vi "SPAN LIN speichern Parameter bestimmern.vi"(11 "SpanInletClusterArray out (Eingang)":T1[](array[typedef]) {"zusätzliche Zeitdauer Erster Punkt" min=30 step=1 format="%#_5g"; "Zeitdauer Stufen" format="%#_5g"; "Max Fehler" format="%#_5g"; "Anzahl Stufen" format="%#_5g"; "Komponenten"."Komponente 5"."Komponente:" items=["NO (350,3000) LP 191C", "NO2 (150) LP 191C (1of2)", "NO2 (2000) LP 191C (2of2)", "N2O (300) LP 191C (1of2)", "NH3 (300) LP 191C (1of2)", "NH3 (900,3000) LP 191C (2of2)", "HNCO (400) 191C", "H2O% (30) LP 191C", "Formaldehyde (70,500) LP 191C", "CO2 low% (4) LP 191C (2of2)", "CO2% (20) LP 191C (1of2)", "CO (700) LP 191C (1of3)", "CO% (1) LP 191C (2of3)", "Propylene (1000) LP 191C", "Aromatic HC C7 (500) LP 191C", "Ethylene (1000) LP 191C", "CH4 (250) LP 191C (1of2)", "CH4 (5000) LP 191C (2of2)", "Ethane (1000) LP 191C", "Acetylene (1000) LP 191C", "HNO2 (20) 191C", "MeOH (1000) 191C", "CO% (10) LP 191C (3of3)", "Formic Acid (100) 191C", "SO2 (500) LP 191C", "Acetaldehyde (1000) LP 191C", "COS (100) LP 191C", "1,3 butadiene (100) LP 191C", "Oil as Octane (200) LP 191C", "N2O (1000) LP 191C (2of2)", "Propane (200) LP 191C", "NO2 autorange (2000)", "CO autorange (100000)", "CH4 autorange (5000)", "NH3 autorange (3000)", "Temp. Gascell", "Pressure Gascell", "sBeam@2500"]; "Komponenten"."Komponente 5"."Konzentration IST" format="%#.4f"; "Komponenten"."Komponente 5"."Genauigkeit" format="%#.1f"; "Komponenten"."Komponente 4"."Komponente:" items=["NO (350,3000) LP 191C", "NO2 (150) LP 191C (1of2)", "NO2 (2000) LP 191C (2of2)", "N2O (300) LP 191C (1of2)", "NH3 (300) LP 191C (1of2)", "NH3 (900,3000) LP 191C (2of2)", "HNCO (400) 191C", "H2O% (30) LP 191C", "Formaldehyde (70,500) LP 191C", "CO2 low% (4) LP 191C (2of2)", "CO2% (20) LP 191C (1of2)", "CO (700) LP 191C (1of3)", "CO% (1) LP 191C (2of3)", "Propylene (1000) LP 191C", "Aromatic HC C7 (500) LP 191C", "Ethylene (1000) LP 191C", "CH4 (250) LP 191C (1of2)", "CH4 (5000) LP 191C (2of2)", "Ethane (1000) LP 191C", "Acetylene (1000) LP 191C", "HNO2 (20) 191C", "MeOH (1000) 191C", "CO% (10) LP 191C (3of3)", "Formic Acid (100) 191C", "SO2 (500) LP 191C", "Acetaldehyde (1000) LP 191C", "COS (100) LP 191C", "1,3 butadiene (100) LP 191C", "Oil as Octane (200) LP 191C", "N2O (1000) LP 191C (2of2)", "Propane (200) LP 191C", "NO2 autorange (2000)", "CO autorange (100000)", "CH4 autorange (5000)", "NH3 autorange (3000)", "Temp. Gascell", "Pressure Gascell", "sBeam@2500"]; "Komponenten"."Komponente 4"."Konzentration IST" format="%#.4f"; "Komponenten"."Komponente 4"."Genauigkeit" format="%#.1f"; "Komponenten"."Komponente 3"."Komponente:" items=["NO (350,3000) LP 191C", "NO2 (150) LP 191C (1of2)", "NO2 (2000) LP 191C (2of2)", "N2O (300) LP 191C (1of2)", "NH3 (300) LP 191C (1of2)", "NH3 (900,3000) LP 191C (2of2)", "HNCO (400) 191C", "H2O% (30) LP 191C", "Formaldehyde (70,500) LP 191C", "CO2 low% (4) LP 191C (2of2)", "CO2% (20) LP 191C (1of2)", "CO (700) LP 191C (1of3)", "CO% (1) LP 191C (2of3)", "Propylene (1000) LP 191C", "Aromatic HC C7 (500) LP 191C", "Ethylene (1000) LP 191C", "CH4 (250) LP 191C (1of2)", "CH4 (5000) LP 191C (2of2)", "Ethane (1000) LP 191C", "Acetylene (1000) LP 191C", "HNO2 (20) 191C", "MeOH (1000) 191C", "CO% (10) LP 191C (3of3)", "Formic Acid (100) 191C", "SO2 (500) LP 191C", "Acetaldehyde (1000) LP 191C", "COS (100) LP 191C", "1,3 butadiene (100) LP 191C", "Oil as Octane (200) LP 191C", "N2O (1000) LP 191C (2of2)", "Propane (200) LP 191C", "NO2 autorange (2000)", "CO autorange (100000)", "CH4 autorange (5000)", "NH3 autorange (3000)", "Temp. Gascell", "Pressure Gascell", "sBeam@2500"]; "Komponenten"."Komponente 3"."Konzentration IST" format="%#.4f"; "Komponenten"."Komponente 3"."Genauigkeit" format="%#.1f"; "Komponenten"."Komponente 2"."Komponente:" items=["NO (350,3000) LP 191C", "NO2 (150) LP 191C (1of2)", "NO2 (2000) LP 191C (2of2)", "N2O (300) LP 191C (1of2)", "NH3 (300) LP 191C (1of2)", "NH3 (900,3000) LP 191C (2of2)", "HNCO (400) 191C", "H2O% (30) LP 191C", "Formaldehyde (70,500) LP 191C", "CO2 low% (4) LP 191C (2of2)", "CO2% (20) LP 191C (1of2)", "CO (700) LP 191C (1of3)", "CO% (1) LP 191C (2of3)", "Propylene (1000) LP 191C", "Aromatic HC C7 (500) LP 191C", "Ethylene (1000) LP 191C", "CH4 (250) LP 191C (1of2)", "CH4 (5000) LP 191C (2of2)", "Ethane (1000) LP 191C", "Acetylene (1000) LP 191C", "HNO2 (20) 191C", "MeOH (1000) 191C", "CO% (10) LP 191C (3of3)", "Formic Acid (100) 191C", "SO2 (500) LP 191C", "Acetaldehyde (1000) LP 191C", "COS (100) LP 191C", "1,3 butadiene (100) LP 191C", "Oil as Octane (200) LP 191C", "N2O (1000) LP 191C (2of2)", "Propane (200) LP 191C", "NO2 autorange (2000)", "CO autorange (100000)", "CH4 autorange (5000)", "NH3 autorange (3000)", "Temp. Gascell", "Pressure Gascell", "sBeam@2500"]; "Komponenten"."Komponente 2"."Konzentration IST" format="%#.4f"; "Komponenten"."Komponente 2"."Genauigkeit" format="%#.1f"; "Komponenten"."Komponente 1"."Komponente:" items=["NO (350,3000) LP 191C", "NO2 (150) LP 191C (1of2)", "NO2 (2000) LP 191C (2of2)", "N2O (300) LP 191C (1of2)", "NH3 (300) LP 191C (1of2)", "NH3 (900,3000) LP 191C (2of2)", "HNCO (400) 191C", "H2O% (30) LP 191C", "Formaldehyde (70,500) LP 191C", "CO2 low% (4) LP 191C (2of2)", "CO2% (20) LP 191C (1of2)", "CO (700) LP 191C (1of3)", "CO% (1) LP 191C (2of3)", "Propylene (1000) LP 191C", "Aromatic HC C7 (500) LP 191C", "Ethylene (1000) LP 191C", "CH4 (250) LP 191C (1of2)", "CH4 (5000) LP 191C (2of2)", "Ethane (1000) LP 191C", "Acetylene (1000) LP 191C", "HNO2 (20) 191C", "MeOH (1000) 191C", "CO% (10) LP 191C (3of3)", "Formic Acid (100) 191C", "SO2 (500) LP 191C", "Acetaldehyde (1000) LP 191C", "COS (100) LP 191C", "1,3 butadiene (100) LP 191C", "Oil as Octane (200) LP 191C", "N2O (1000) LP 191C (2of2)", "Propane (200) LP 191C", "NO2 autorange (2000)", "CO autorange (100000)", "CH4 autorange (5000)", "NH3 autorange (3000)", "Temp. Gascell", "Pressure Gascell", "sBeam@2500"]; "Komponenten"."Komponente 1"."Konzentration IST" format="%#.4f"; "Komponenten"."Komponente 1"."Genauigkeit" format="%#.1f"; "Ablaufdatum" format="%<%d.%m.%Y>T"; "Gasflasche" items=["----"=10000, "IAG NH3 3000"=0, "IAG NH3 200"=1, "IAG NH3 2000"=2, "IAG MG"=3, "IAG O2"=4]}) -> (0 "Anzahl Komponenten OK":bool, 1 "gültige aktiver auto SPAN Index":bool, 2 "Anzahl aktive Komponenten out":i32, 3 "SpanInletClusterArray out (Ausgang)":T1[](array[typedef]) {"zusätzliche Zeitdauer Erster Punkt" min=30 step=1 format="%#_5g"; "Zeitdauer Stufen" format="%#_5g"; "Max Fehler" format="%#_5g"; "Anzahl Stufen" format="%#_5g"; "Komponenten"."Komponente 5"."Komponente:" items=["NO (350,3000) LP 191C", "NO2 (150) LP 191C (1of2)", "NO2 (2000) LP 191C (2of2)", "N2O (300) LP 191C (1of2)", "NH3 (300) LP 191C (1of2)", "NH3 (900,3000) LP 191C (2of2)", "HNCO (400) 191C", "H2O% (30) LP 191C", "Formaldehyde (70,500) LP 191C", "CO2 low% (4) LP 191C (2of2)", "CO2% (20) LP 191C (1of2)", "CO (700) LP 191C (1of3)", "CO% (1) LP 191C (2of3)", "Propylene (1000) LP 191C", "Aromatic HC C7 (500) LP 191C", "Ethylene (1000) LP 191C", "CH4 (250) LP 191C (1of2)", "CH4 (5000) LP 191C (2of2)", "Ethane (1000) LP 191C", "Acetylene (1000) LP 191C", "HNO2 (20) 191C", "MeOH (1000) 191C", "CO% (10) LP 191C (3of3)", "Formic Acid (100) 191C", "SO2 (500) LP 191C", "Acetaldehyde (1000) LP 191C", "COS (100) LP 191C", "1,3 butadiene (100) LP 191C", "Oil as Octane (200) LP 191C", "N2O (1000) LP 191C (2of2)", "Propane (200) LP 191C", "NO2 autorange (2000)", "CO autorange (100000)", "CH4 autorange (5000)", "NH3 autorange (3000)", "Temp. Gascell", "Pressure Gascell", "sBeam@2500"]; "Komponenten"."Komponente 5"."Konzentration IST" format="%#.4f"; "Komponenten"."Komponente 5"."Genauigkeit" format="%#.1f"; "Komponenten"."Komponente 4"."Komponente:" items=["NO (350,3000) LP 191C", "NO2 (150) LP 191C (1of2)", "NO2 (2000) LP 191C (2of2)", "N2O (300) LP 191C (1of2)", "NH3 (300) LP 191C (1of2)", "NH3 (900,3000) LP 191C (2of2)", "HNCO (400) 191C", "H2O% (30) LP 191C", "Formaldehyde (70,500) LP 191C", "CO2 low% (4) LP 191C (2of2)", "CO2% (20) LP 191C (1of2)", "CO (700) LP 191C (1of3)", "CO% (1) LP 191C (2of3)", "Propylene (1000) LP 191C", "Aromatic HC C7 (500) LP 191C", "Ethylene (1000) LP 191C", "CH4 (250) LP 191C (1of2)", "CH4 (5000) LP 191C (2of2)", "Ethane (1000) LP 191C", "Acetylene (1000) LP 191C", "HNO2 (20) 191C", "MeOH (1000) 191C", "CO% (10) LP 191C (3of3)", "Formic Acid (100) 191C", "SO2 (500) LP 191C", "Acetaldehyde (1000) LP 191C", "COS (100) LP 191C", "1,3 butadiene (100) LP 191C", "Oil as Octane (200) LP 191C", "N2O (1000) LP 191C (2of2)", "Propane (200) LP 191C", "NO2 autorange (2000)", "CO autorange (100000)", "CH4 autorange (5000)", "NH3 autorange (3000)", "Temp. Gascell", "Pressure Gascell", "sBeam@2500"]; "Komponenten"."Komponente 4"."Konzentration IST" format="%#.4f"; "Komponenten"."Komponente 4"."Genauigkeit" format="%#.1f"; "Komponenten"."Komponente 3"."Komponente:" items=["NO (350,3000) LP 191C", "NO2 (150) LP 191C (1of2)", "NO2 (2000) LP 191C (2of2)", "N2O (300) LP 191C (1of2)", "NH3 (300) LP 191C (1of2)", "NH3 (900,3000) LP 191C (2of2)", "HNCO (400) 191C", "H2O% (30) LP 191C", "Formaldehyde (70,500) LP 191C", "CO2 low% (4) LP 191C (2of2)", "CO2% (20) LP 191C (1of2)", "CO (700) LP 191C (1of3)", "CO% (1) LP 191C (2of3)", "Propylene (1000) LP 191C", "Aromatic HC C7 (500) LP 191C", "Ethylene (1000) LP 191C", "CH4 (250) LP 191C (1of2)", "CH4 (5000) LP 191C (2of2)", "Ethane (1000) LP 191C", "Acetylene (1000) LP 191C", "HNO2 (20) 191C", "MeOH (1000) 191C", "CO% (10) LP 191C (3of3)", "Formic Acid (100) 191C", "SO2 (500) LP 191C", "Acetaldehyde (1000) LP 191C", "COS (100) LP 191C", "1,3 butadiene (100) LP 191C", "Oil as Octane (200) LP 191C", "N2O (1000) LP 191C (2of2)", "Propane (200) LP 191C", "NO2 autorange (2000)", "CO autorange (100000)", "CH4 autorange (5000)", "NH3 autorange (3000)", "Temp. Gascell", "Pressure Gascell", "sBeam@2500"]; "Komponenten"."Komponente 3"."Konzentration IST" format="%#.4f"; "Komponenten"."Komponente 3"."Genauigkeit" format="%#.1f"; "Komponenten"."Komponente 2"."Komponente:" items=["NO (350,3000) LP 191C", "NO2 (150) LP 191C (1of2)", "NO2 (2000) LP 191C (2of2)", "N2O (300) LP 191C (1of2)", "NH3 (300) LP 191C (1of2)", "NH3 (900,3000) LP 191C (2of2)", "HNCO (400) 191C", "H2O% (30) LP 191C", "Formaldehyde (70,500) LP 191C", "CO2 low% (4) LP 191C (2of2)", "CO2% (20) LP 191C (1of2)", "CO (700) LP 191C (1of3)", "CO% (1) LP 191C (2of3)", "Propylene (1000) LP 191C", "Aromatic HC C7 (500) LP 191C", "Ethylene (1000) LP 191C", "CH4 (250) LP 191C (1of2)", "CH4 (5000) LP 191C (2of2)", "Ethane (1000) LP 191C", "Acetylene (1000) LP 191C", "HNO2 (20) 191C", "MeOH (1000) 191C", "CO% (10) LP 191C (3of3)", "Formic Acid (100) 191C", "SO2 (500) LP 191C", "Acetaldehyde (1000) LP 191C", "COS (100) LP 191C", "1,3 butadiene (100) LP 191C", "Oil as Octane (200) LP 191C", "N2O (1000) LP 191C (2of2)", "Propane (200) LP 191C", "NO2 autorange (2000)", "CO autorange (100000)", "CH4 autorange (5000)", "NH3 autorange (3000)", "Temp. Gascell", "Pressure Gascell", "sBeam@2500"]; "Komponenten"."Komponente 2"."Konzentration IST" format="%#.4f"; "Komponenten"."Komponente 2"."Genauigkeit" format="%#.1f"; "Komponenten"."Komponente 1"."Komponente:" items=["NO (350,3000) LP 191C", "NO2 (150) LP 191C (1of2)", "NO2 (2000) LP 191C (2of2)", "N2O (300) LP 191C (1of2)", "NH3 (300) LP 191C (1of2)", "NH3 (900,3000) LP 191C (2of2)", "HNCO (400) 191C", "H2O% (30) LP 191C", "Formaldehyde (70,500) LP 191C", "CO2 low% (4) LP 191C (2of2)", "CO2% (20) LP 191C (1of2)", "CO (700) LP 191C (1of3)", "CO% (1) LP 191C (2of3)", "Propylene (1000) LP 191C", "Aromatic HC C7 (500) LP 191C", "Ethylene (1000) LP 191C", "CH4 (250) LP 191C (1of2)", "CH4 (5000) LP 191C (2of2)", "Ethane (1000) LP 191C", "Acetylene (1000) LP 191C", "HNO2 (20) 191C", "MeOH (1000) 191C", "CO% (10) LP 191C (3of3)", "Formic Acid (100) 191C", "SO2 (500) LP 191C", "Acetaldehyde (1000) LP 191C", "COS (100) LP 191C", "1,3 butadiene (100) LP 191C", "Oil as Octane (200) LP 191C", "N2O (1000) LP 191C (2of2)", "Propane (200) LP 191C", "NO2 autorange (2000)", "CO autorange (100000)", "CH4 autorange (5000)", "NH3 autorange (3000)", "Temp. Gascell", "Pressure Gascell", "sBeam@2500"]; "Komponenten"."Komponente 1"."Konzentration IST" format="%#.4f"; "Komponenten"."Komponente 1"."Genauigkeit" format="%#.1f"; "Ablaufdatum" format="%<%d.%m.%Y>T"; "Gasflasche" items=["----"=10000, "IAG NH3 3000"=0, "IAG NH3 200"=1, "IAG NH3 2000"=2, "IAG MG"=3, "IAG O2"=4]}, 4 "Zeitstempel":timestamp, 5 "Anzahl Namen":i32, 6 "Component Infos":T10, 7 "postprocess":bool, 8 "PDF start":bool)   [LabVIEW 2020, in "Linearisierung v2.lvlib" / "SpanEinstellungen.lvlib"]
uses:
  SpanEinstellungen.lvlib
  SpanInletCluster.ctl
  Seiten/System Einstellungen V2/Konfig Gasflasche.ctl
  Seiten/System Einstellungen V2/Analysatoren.ctl
  Seiten/System Einstellungen V2/Gasflasche Auswahl.ctl
  Komponentencluster mit Formel.ctl
  Komponentenauswahl mit Formel.ctl
  Visualisierungs Elemente/String - Eingabefeld.ctl
  Einheit.ctl
  Seiten/System Einstellungen V2/Traegergas.ctl
  ComponentInfos.ctl
  Visualisierungs Elemente/String - Ausgabefeld.ctl
  Aktion FGV Spans abarbeiten.ctl
  Aktion FGV Post Processing.ctl
  Aktion FGV SPAN Verriegelung.ctl
  Seiten/System Einstellungen V2/System Einstellungen V2.lvlib
panel:
  # "sec"
  # "%"
  # "sec"
  # "Komponente"
  # "Formel"
  # "Konzentration"
  # "Einheit"
  # "Genauigkeit [%]"
  # "sec"
  # "%"
  # "sec"
  # "Komponente"
  # "Formel"
  # "Konzentration"
  # "Einheit"
  # "Genauigkeit [%]"
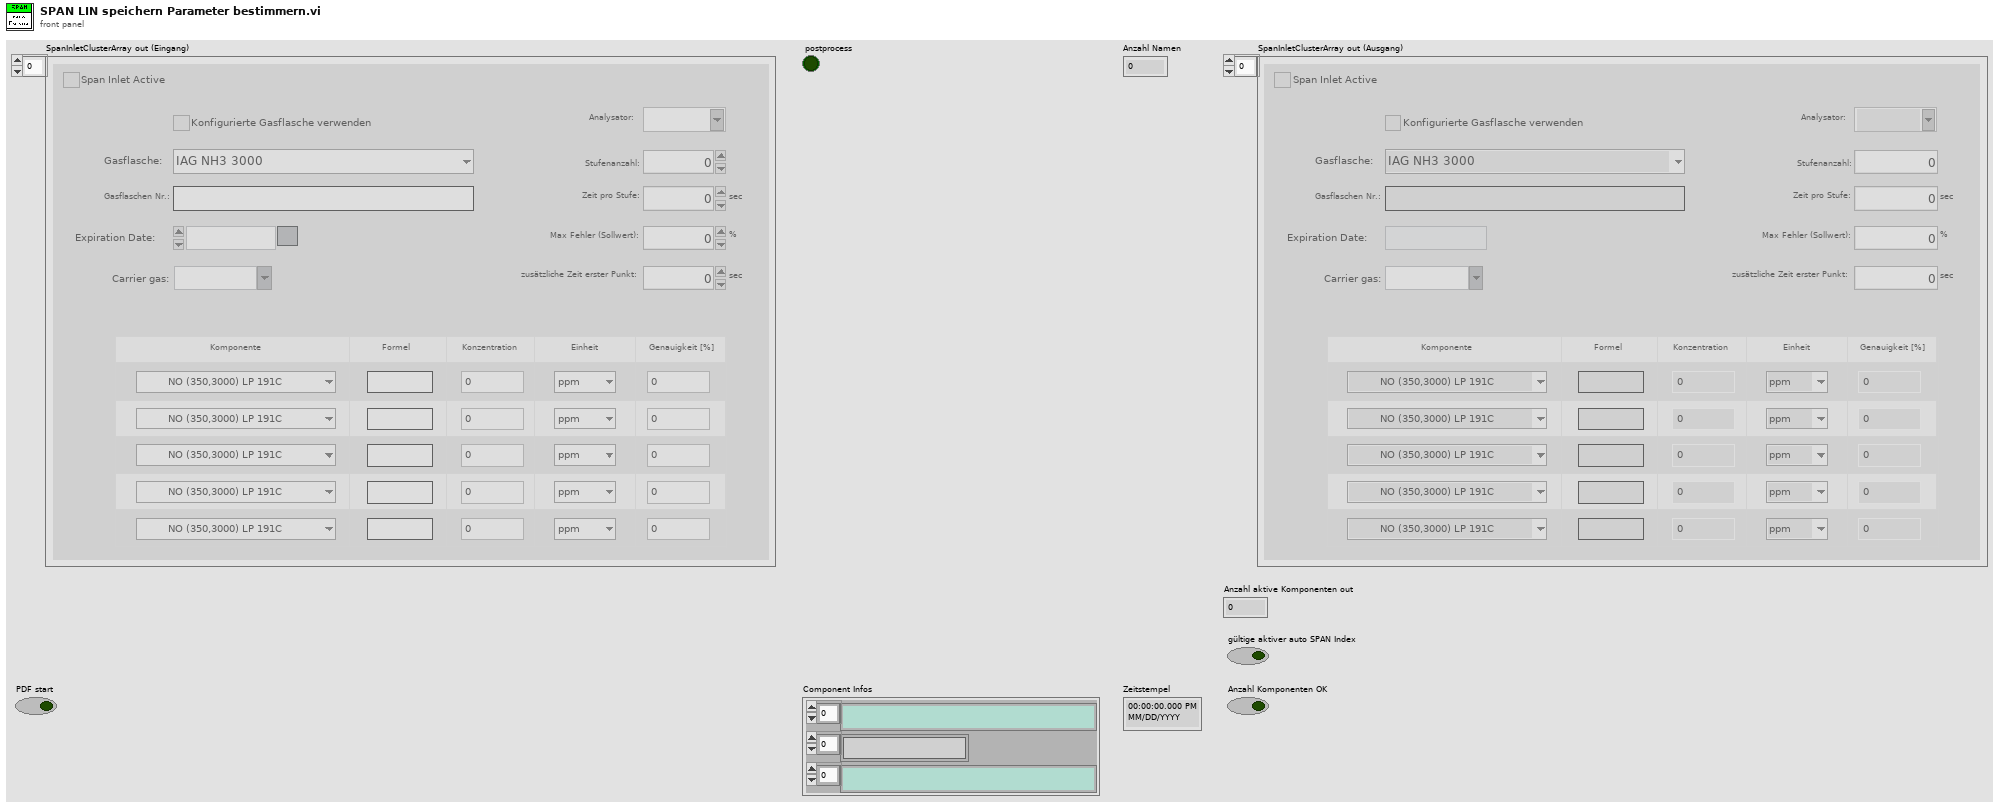
[diagram p1: front panel]
types:
  T1 = typedef "Linearisierung v2.lvlib/SpanEinstellungen.lvlib/SpanInletCluster.ctl" = cluster{"Span Inlet Active":T2, "Analysator":T3, "Konfig Gasflasche":T2, "Gasflasche":T4, "Gasflaschen Nr.:":string, "Ablaufdatum":timestamp, "Komponenten":T5, "Zeitdauer Stufen":sgl, "Max Fehler":sgl, "Anzahl Stufen":sgl, "Trägergas":T9, "zusätzliche Zeitdauer Erster Punkt":sgl}
  T2 = typedef "System Einstellungen V2.lvlib/Konfig Gasflasche.ctl" = bool
  T3 = typedef "System Einstellungen V2.lvlib/Analysatoren.ctl" = string
  T4 = typedef "System Einstellungen V2.lvlib/Gasflasche Auswahl.ctl" = u16
  T5 = typedef "Linearisierung v2.lvlib/SpanEinstellungen.lvlib/Komponentencluster mit Formel.ctl" = cluster{"Komponente 1":T6, "Komponente 2":T6, "Komponente 3":T6, "Komponente 4":T6, "Komponente 5":T6}
  T6 = typedef "Linearisierung v2.lvlib/SpanEinstellungen.lvlib/Komponentenauswahl mit Formel.ctl" = cluster{"Komponente:":u16, "Summenformel":T7, "Konzentration IST":dbl, "Einheit":T8, "Genauigkeit":dbl}
  T7 = typedef "String - Eingabefeld.ctl" = string
  T8 = typedef "Linearisierung v2.lvlib/SpanEinstellungen.lvlib/Einheit.ctl" = enum16{"ppm", "%"}
  T9 = typedef "System Einstellungen V2.lvlib/Traegergas.ctl" = string
  T10 = typedef "Linearisierung v2.lvlib/SpanEinstellungen.lvlib/ComponentInfos.ctl" = cluster{T11[], T7[], T11[]}
  T11 = typedef "String - Ausgabefeld.ctl" = string
  T12 = typedef "Linearisierung v2.lvlib/SpanEinstellungen.lvlib/Aktion FGV Spans abarbeiten.ctl" = enum16{"lesen", "idle", "start", "next", "comp", "init", "running", "abort"}
  T13 = typedef "Linearisierung v2.lvlib/SpanEinstellungen.lvlib/Aktion FGV SPAN Verriegelung.ctl" = enum16{"lesen", "setrefs", "setcomp", "lock", "unlock", "Set Save EPA redirect", "Reset Save EPA redirect", "Set Postprocessing PDF", "Reset Postprocessing PDF", "Set Start Postprocessing PDF", "Reset Start Postprocessing PDF"}
  T14 = typedef "Linearisierung v2.lvlib/SpanEinstellungen.lvlib/Aktion FGV Post Processing.ctl" = enum16{"lesen", "set ref", "init", "reset", "enable", "disable", "filenames", "active", "comp", "filename index", "next", "first", "abort", "show"}
  T15 = typedef "Linearisierung v2.lvlib/SpanEinstellungen.lvlib/Postprocessing_Running_Indices.ctl" = cluster{"active postprocessing SPAN":i32, "active postprocessing SPAN Component":i32, "active postprocessing index":i32}
  T16 = cluster{"active Index Cluster out":T15, "last postprocessing SPAN ":bool}
  T17 = cluster{"locked":bool, "Save EPA redirect":bool, "Postprocessing PDF":bool, "Start Postprocessing PDF":bool}
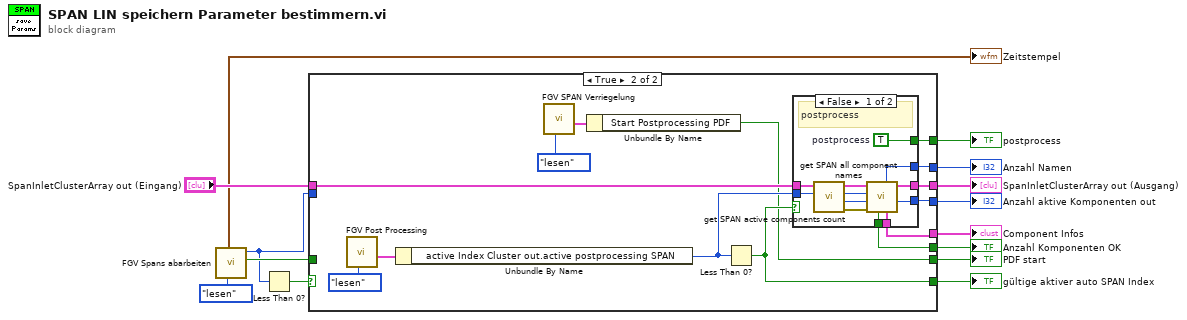
[diagram p0: block diagram]
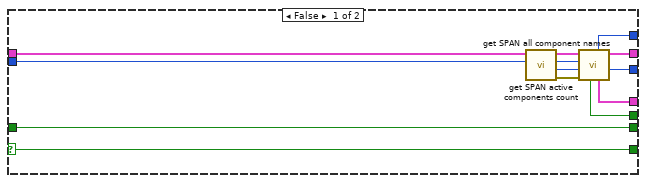
[diagram p2: hidden frame]
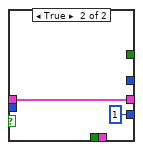
[diagram p3: hidden frame]
diagram:
  n1 = call "FGV Spans abarbeiten.vi"("Aktion"=Aktion_FGV_Spans_abarbeiten."lesen") -> ("start"=w12:bool, "active SPAN Idx out"=w10:i32, "Zeitstempel"=→"Zeitstempel":timestamp)  [unwired: 5 in, 3 out]
  n2 = Less Than 0?(x=w10) -> (x < 0?=w11:bool)
  n3 = case shown="True" w11 {
    selector: w11 -> [w15 _]
    tunnel: w10 -> [w27 _]
    tunnel: "SpanInletClusterArray out (Eingang)" -> [w26 w38]
    tunnel: [w22 w40] -> w6
    tunnel: [w20 w34] -> w7
    tunnel: [w19 w33] -> w8
    tunnel: [w18 w35] -> w9
    tunnel: w12 -> [w16 _]
    tunnel: [w16 w28] -> w13
    tunnel: [w15 w39] -> w14
    tunnel: [w17 w37] -> w2
    tunnel: [_ w32] -> w1
    frame False {
      n4 = call "get SPAN active components count.vi"("SPAN Idx"=w27, "SpanInletClusterArray in"=w26) -> ("error out"=w21:errorcluster, "Anzahl aktive Komponenten"=w23:i32, "SPAN Idx out"=w24:i32, "SpanInletClusterArray out"=w25:T1[])  [unwired: 6 in]
      n5 = call "get SPAN all component names.vi"("error in (no error)"=w21, "Anzahl aktive Komponenten"=w23, "active SPAN Idx"=w24, "SpanInletClusterArray in"=w25) -> ("Anzahl aktive Komponenten out"=w22:i32, "SpanInletClusterArray out"=w17:T1[], "Component Infos"=w20:T10, "Anzahl Namen"=w18:i32, "OK"=w19:bool)  [unwired: 1 in, 2 out]
    }
    frame True {
      n6 = call "FGV Post Processing.vi"("Aktion"=Aktion_FGV_Post_Processing."lesen") -> ("active Index Cluster out"=w36:T16)  [unwired: 7 in, 3 out]
      n7 = Unbundle By Name(w36) -> ("active Index Cluster out.active postprocessing SPAN"=w31:i32)
      n8 = call "FGV SPAN Verriegelung.vi"("aktion"=Aktion_FGV_SPAN_Verriegelung."lesen") -> ("Flags Cluster"=w29:T17)  [unwired: 8 in, 2 out]
      n9 = Unbundle By Name(w29) -> ("Start Postprocessing PDF"=w28:bool)
      n10 = Less Than 0?(x=w31) -> (x < 0?=w39:bool)
      n11 = case shown="False" w39 {
        tunnel: [w46 1 ("Anzahl aktive Komponenten out")] -> w40
        tunnel: w38 -> [w49 w54]
        tunnel: [w48 w54] -> w37
        tunnel: w31 -> [w47 _]
        tunnel: [w45 _] -> w35
        tunnel: [w44 _] -> w34
        tunnel: [w43 _] -> w33
        tunnel: [w42 _] -> w32
        frame False {
          w42 = TRUE  # postprocess
          # "postprocess"
          n12 = call "get SPAN active components count.vi"("SPAN Idx"=w47, "SpanInletClusterArray in"=w49) -> ("error out"=w50:errorcluster, "Anzahl aktive Komponenten"=w51:i32, "SPAN Idx out"=w52:i32, "SpanInletClusterArray out"=w53:T1[])  [unwired: 6 in]
          n13 = call "get SPAN all component names.vi"("error in (no error)"=w50, "Anzahl aktive Komponenten"=w51, "active SPAN Idx"=w52, "SpanInletClusterArray in"=w53) -> ("Anzahl aktive Komponenten out"=w46:i32, "SpanInletClusterArray out"=w48:T1[], "Component Infos"=w44:T10, "Anzahl Namen"=w45:i32, "OK"=w43:bool)  [unwired: 1 in, 2 out]
        }
        frame True {
        }
      }
    }
  }
  "gültige aktiver auto SPAN Index" <- w14
  "PDF start" <- w13
  "SpanInletClusterArray out (Ausgang)" <- w2
  "Anzahl Namen" <- w9
  "Anzahl Komponenten OK" <- w8
  "Component Infos" <- w7
  "Anzahl aktive Komponenten out" <- w6
  "postprocess" <- w1
